vi "AV Write Array.vi"(8 "error in":errorcluster, 10 "Humidity AV":dbl[](array[numeric]), 11 "Pressure Actual Value in":refnum<class "Pressure Actual Value.lvclass">) -> (0 "error out":errorcluster, 3 "Pressure Actual Value out":refnum<class "Pressure Actual Value.lvclass">)   [LabVIEW 2023, in "Pressure Actual Value.lvclass"]
uses:
  Pressure Actual Value.lvclass
  Parents/Actual Value/Actual Value.lvclass
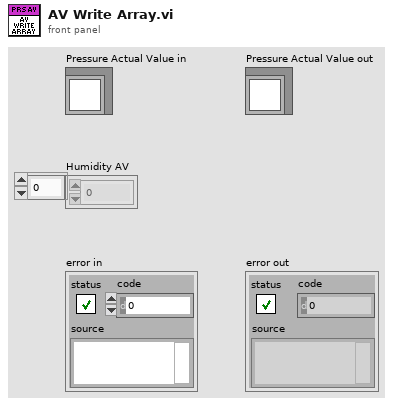
[diagram p1: front panel]
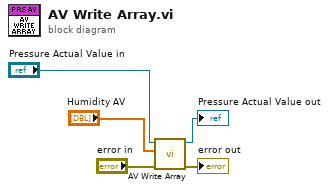
[diagram p0: block diagram]
diagram:
  n1 = call-parent "AV Write Array.vi"("error in"="error in", "Actual Value"="Humidity AV", "Actual Value in"="Pressure Actual Value in") -> ("error out"=→"error out":errorcluster, "Actual Value out"=→"Pressure Actual Value out":refnum<class "Pressure Actual Value.lvclass">)  [unwired: 7 in]
